vi "Get Username.vi"(8 "error in (no error)":errorcluster, 11 "RT Management Session in":refnum<class "RT Management.lvclass">) -> (0 "error out":errorcluster, 2 "Username":string, 3 "RT Management Session out":refnum<class "RT Management.lvclass">)   [LabVIEW 2016, in "RT Management.lvlib" / "RT Management.lvclass"]
uses:
  RT Management.lvclass
  RT Management.lvclass/RT Management.ctl
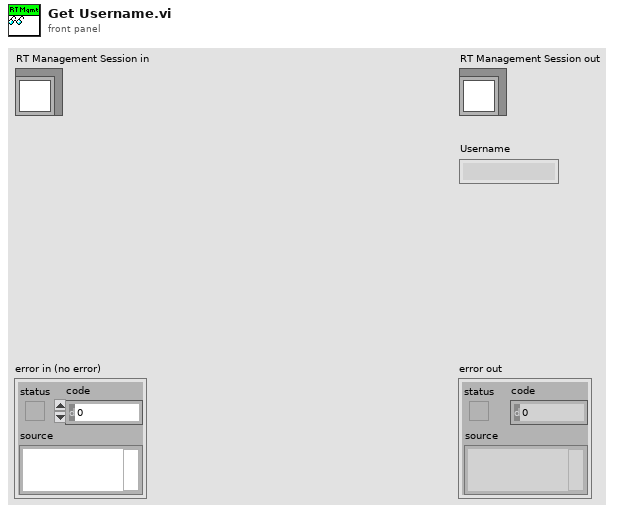
[diagram p1: front panel]
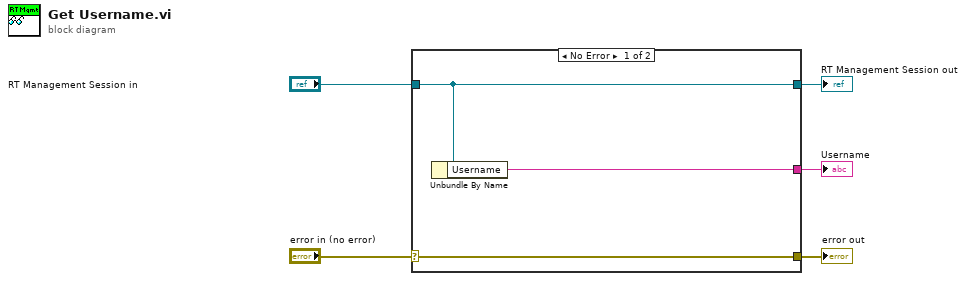
[diagram p0: block diagram]
diagram:
  n1 = case shown="No Error" "error in (no error)" {
    selector: "error in (no error)" -> [w8 w9]
    tunnel: [w8 w9] -> w4
    tunnel: [w7 w10] -> w2
    tunnel: "RT Management Session in" -> [w7 w10]
    tunnel: [w6 _] -> w1
    frame No Error {
      n2 = Unbundle By Name(w7) -> ("Username"=w6:string)
    }
    frame Error {
    }
  }
  "error out" <- w4
  "RT Management Session out" <- w2
  "Username" <- w1
